vi "Write NF Freq (MHz).vi"(8 "error in (no error)":errorcluster, 10 "NF Freq (MHz)":string, 11 "NF in":refnum<class "NF Eval.lvclass">) -> (0 "error out":errorcluster, 3 "NF out":refnum<class "NF Eval.lvclass">)   [LabVIEW 2016, in "SeqAuto Evaluations.lvlib" / "NF Eval.lvclass"]
uses:
  NF Eval.lvclass
  NF Eval.lvclass/NF Eval.ctl
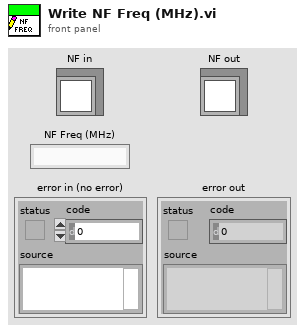
[diagram p1: front panel]
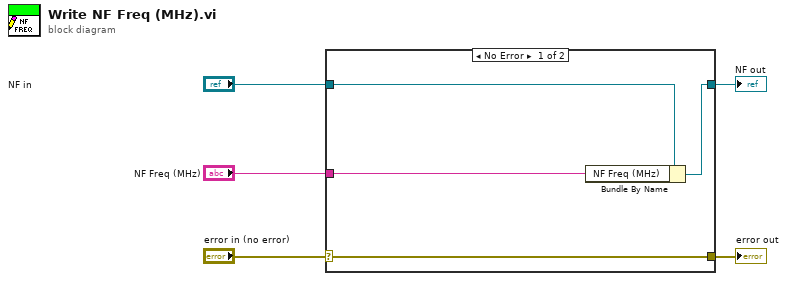
[diagram p0: block diagram]
diagram:
  n1 = case shown="No Error" "error in (no error)" {
    selector: "error in (no error)" -> [w9 w10]
    tunnel: [w9 w10] -> w4
    tunnel: [w7 w11] -> w2
    tunnel: "NF in" -> [w8 w11]
    tunnel: "NF Freq (MHz)" -> [w6 _]
    frame No Error {
      n2 = Bundle By Name(cluster=w8, "NF Freq (MHz)"=w6) -> (w7:refnum<class "NF Eval.lvclass">)
    }
    frame Error {
    }
  }
  "error out" <- w4
  "NF out" <- w2
